vi "Array and MAth operations.vi"() -> ()   [LabVIEW 2024]
uses:
  <vilib>/Analysis/5stat.llb/RMS (DBL).vi
  <vilib>/Analysis/baseanly.llb/Mean (DBL).vi
  <vilib>/Analysis/NI_AALBase.lvlib
  <vilib>/gmath/NI_Gmath.lvlib
  <vilib>/Analysis/NI_AALPro.lvlib
panel:
  in  "Tab Control":T1(tab)
  out "median":dbl format="%0.2f"
  out "error":i32
  out "mean":dbl format="%0.2f"
  out "error 3":i32
  in  "type":T2(ring)
  in  "percent (trim)":dbl=25.0
  out "error 4":i32
  out "mean value":dbl
  in  "Weighting (Sample)":enum16{"Sample", "Population"}(ring)
  out "variance":dbl format="%0.2f"
  out "mean 2":dbl format="%0.2f"
  out "standard deviation":dbl format="%0.2f"
  out "rms value":dbl format="%0.2f"
  out "error 2":i32
  out "error 5":i32
  out "mse":dbl format="%0.2f"
  in  "X Values":dbl[](array[numeric]) format="%0.2f"
  in  "Array":dbl[](array[numeric])
  # "Overview: In this VI, we are practising the use of Arrays and performing some mean operations like man, median, and mode.\nInstructions:\n1. Numerics->Data Containers->Arrays"
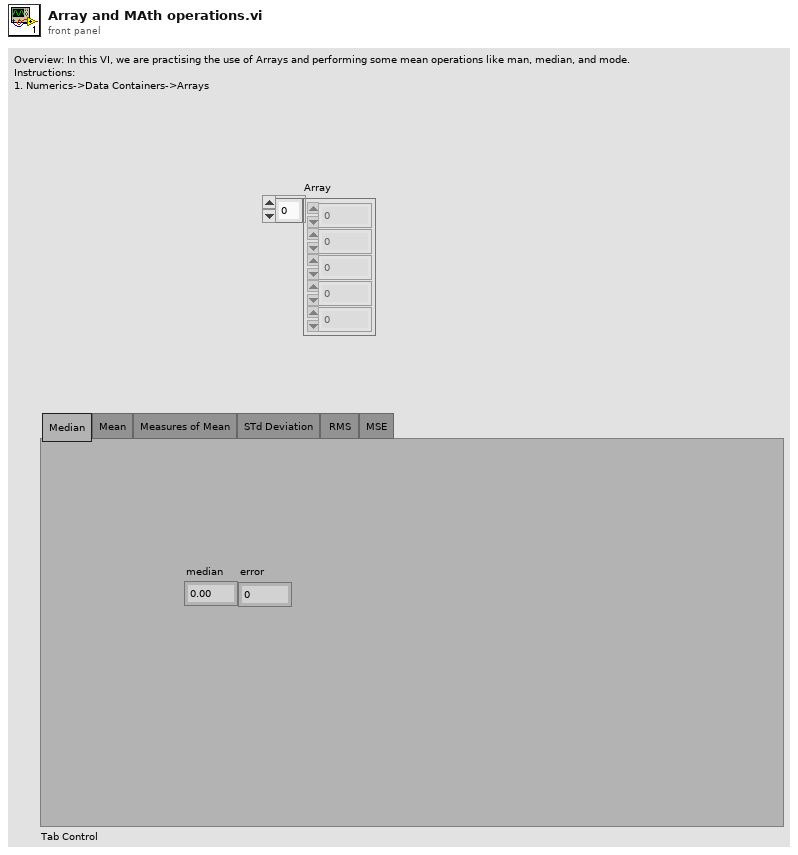
[diagram p1: front panel]
types:
  T1 = enum32{"Median", "Mean", "Measures of Mean", "STd Deviation", "RMS ", "MSE"}
  T2 = enum16{"arithmetic", "geometric", "harmonic", "trimmed", "median"}
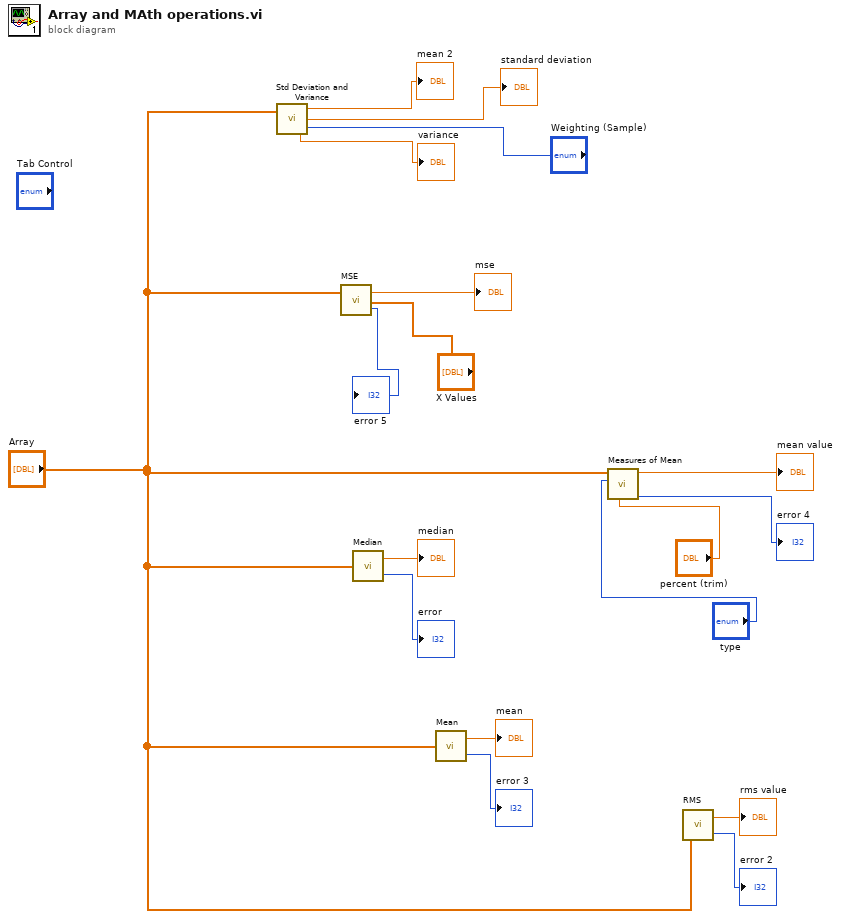
[diagram p0: block diagram]
diagram:
  n1 = call <vilib>:"Std Deviation and Variance.vi"("X"="Array", "Weighting (Sample)"="Weighting (Sample)") -> ("mean"=→"mean 2":dbl, "standard deviation"=→"standard deviation":dbl, "variance"=→"variance":dbl)
  n2 = call <vilib>:"MSE.vi"("X Values"="X Values", "Y Values"="Array") -> ("error"=→"error 5":i32, "mse"=→"mse":dbl)
  n3 = call <vilib>:"Median.vi"("X"="Array") -> ("median"=→"median":dbl, "error"=→"error":i32)
  n4 = call-poly <vilib>:"Mean.vi"("X"="Array") -> ("mean"=→"mean":dbl, "error"=→"error 3":i32)
  n5 = call <vilib>:"Measures of Mean.vi"("percent (trim)"="percent (trim)", "type"="type", "x array"="Array") -> ("error"=→"error 4":i32, "mean value"=→"mean value":dbl)  [unwired: 7 in]
  n6 = call-poly <vilib>:"RMS.vi"("X"="Array") -> ("rms value"=→"rms value":dbl, "error"=→"error 2":i32)
